vi "SCC-manual.vi"() -> (0 "vacuo 2":bool, 1 "vacuo (mBar)":dbl(knob) scale=0.0..1000.0, 2 "P02 (Bar)":dbl(knob) scale=0.0..20.0 scale format="%#_5g", 3 "P01 (Bar)":dbl(knob) scale=0.0..20.0, 4 "ATM 2":bool, 5 "Cam01 2":bool, 6 "Cam02 2":bool, 7 "Gas2":bool, 8 "T-02":dbl, 9 "T-01":dbl, 10 "Tc":dbl, 11 "Boolean":bool)   [LabVIEW 2011]
panel:
  in  "argument 7":dbl
  in  "argument 6":dbl
  in  "argument 5":dbl
  in  "argument 4":dbl
  in  "argument 3":dbl
  in  "argument 2":dbl
  in  "argument":dbl
  in  "Clear":bool
  out "Waveform Chart":T1(graph)
  in  "stop":bool
  out "Heat 2":bool
  out "Pelt 2":bool
  in  "Heat":bool
  in  "Pelt":bool
  in  "vacuo":bool
  in  "Gas":bool
  in  "ATM":bool
  in  "Cam02":bool
  in  "Cam01":bool
  # "Manual controller"
  # "Gas in"
  # "P - 01(bar)"
  # "P - 02(bar)"
  # "Cham-1"
  # "Cham-2"
  # "Atm"
  # "Tc"
  # "T-01"
  # "Vacuo"
  # "T-02"
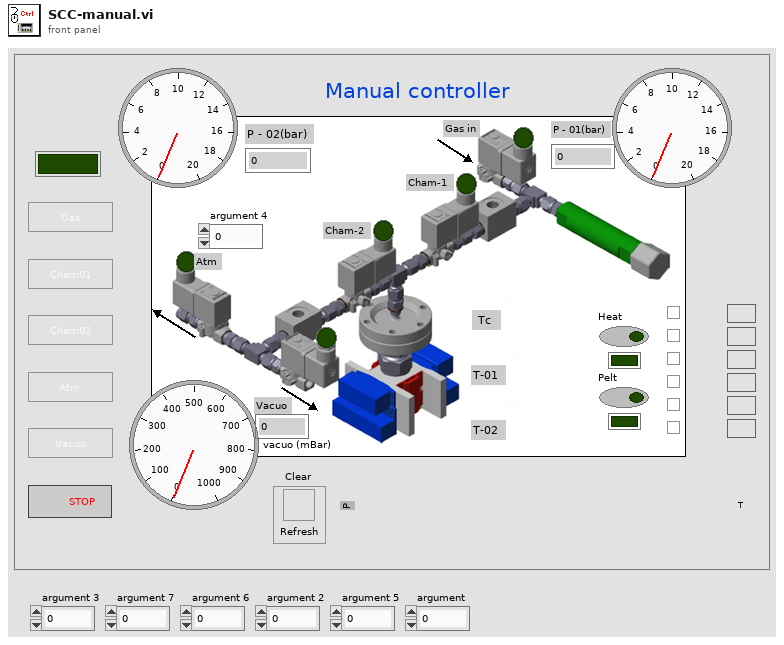
[diagram p1: front panel]
types:
  T1 = cluster{"P01 (Bar)":dbl, "P02 (Bar)":dbl, "vacuo (mBar)":dbl, "RTD-chamber (ºC)":sgl, "RTD-01 (ºC)":sgl, "RTD-02 (ºC)":sgl}
  T2 = cluster{"P01 (Bar)":dbl, "P02 (Bar)":dbl, "vacuo (mBar)":dbl, "RTD-chamber (ºC)":sgl, "RTD-01 (ºC)":sgl, "RTD-02 (ºC)":sgl}[]
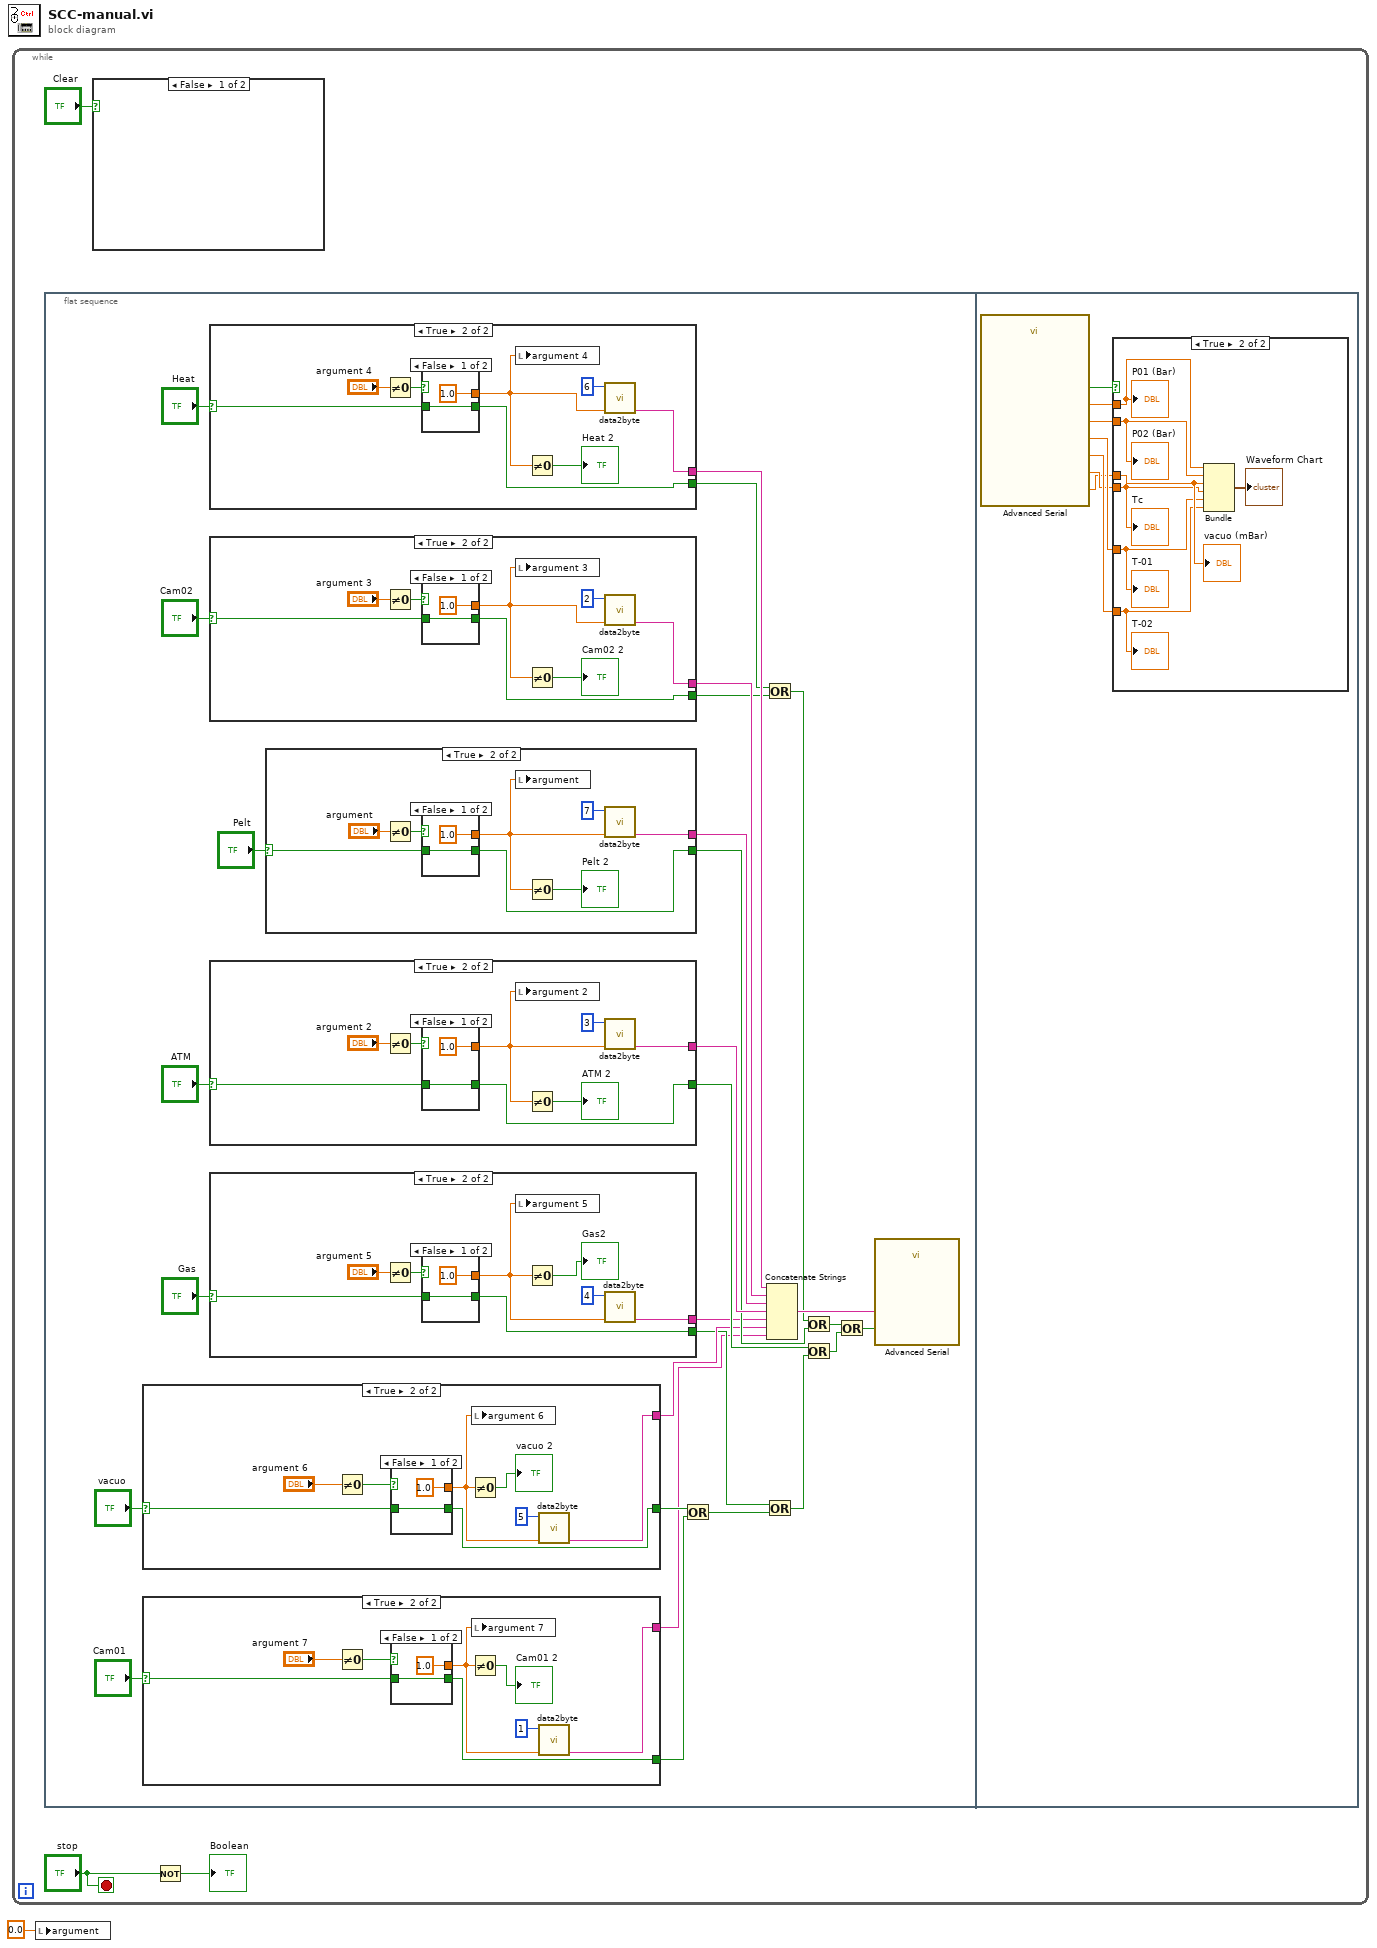
[diagram p0: block diagram]
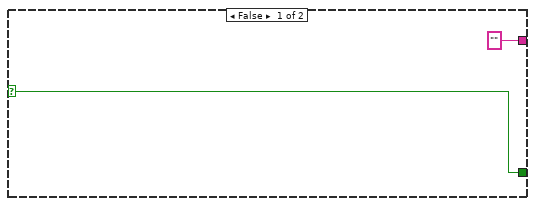
[diagram p2: hidden frame]
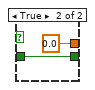
[diagram p3: hidden frame]
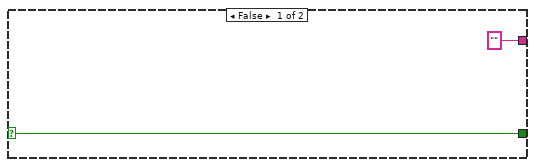
[diagram p4: hidden frame]
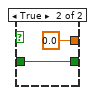
[diagram p5: hidden frame]
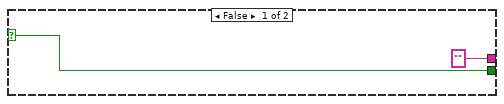
[diagram p6: hidden frame]
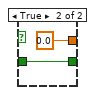
[diagram p7: hidden frame]
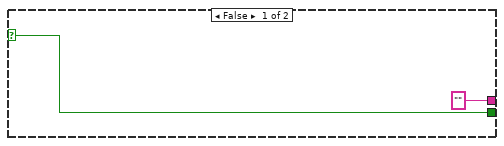
[diagram p8: hidden frame]
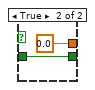
[diagram p9: hidden frame]
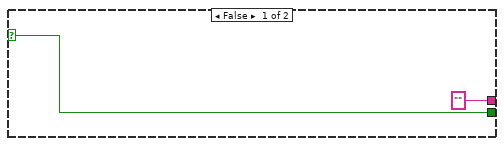
[diagram p10: hidden frame]
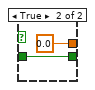
[diagram p11: hidden frame]
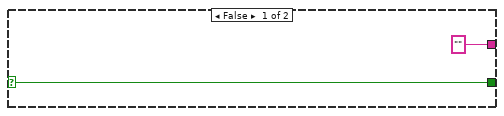
[diagram p12: hidden frame]
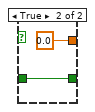
[diagram p13: hidden frame]
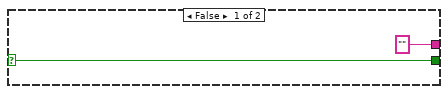
[diagram p14: hidden frame]
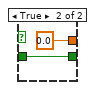
[diagram p15: hidden frame]
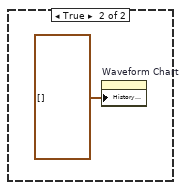
[diagram p17: hidden frame]
diagram:
  n1 = while {
    stop <- "stop" stop-if-true
    n2 = flat-sequence {
      frame #0 {
        n3 = case shown="True" "vacuo" {
          selector: "vacuo" -> [w47 w55]
          tunnel: [w47 w54] -> w7
          tunnel: ["" ("protocol") w50] -> w13
          frame False {
          }
          frame True {
            n4 = Not Equal To 0?(x="argument 6") -> (x != 0?=w56:bool)
            n5 = case shown="False" w56 {
              tunnel: [w58 w60] -> w54
              tunnel: w55 -> [w58 w60]
              tunnel: [1.0 ("number") 0.0 ("number")] -> w51
              frame False {
              }
              frame True {
              }
            }
            n6 = Not Equal To 0?(x=w51) -> (x != 0?=→"vacuo 2":bool)
            n7 = local write "argument 6"(w51) -> ()
            n8 = call "data2byte.vi"("argument"=w51, "new function"=5) -> ("protocol"=w50:string)  [unwired: 8 in, 1 out]
          }
        }
        n9 = case shown="True" "Cam01" {
          selector: "Cam01" -> [w33 w41]
          tunnel: [w33 w40] -> w9
          tunnel: ["" ("protocol") w36] -> w5
          frame False {
          }
          frame True {
            n10 = Not Equal To 0?(x="argument 7") -> (x != 0?=w42:bool)
            n11 = case shown="False" w42 {
              tunnel: [w44 w46] -> w40
              tunnel: w41 -> [w44 w46]
              tunnel: [1.0 ("number") 0.0 ("number")] -> w37
              frame False {
              }
              frame True {
              }
            }
            n12 = Not Equal To 0?(x=w37) -> (x != 0?=→"Cam01 2":bool)
            n13 = local write "argument 7"(w37) -> ()
            n14 = call "data2byte.vi"("argument"=w37, "new function"=1) -> ("protocol"=w36:string)  [unwired: 8 in, 1 out]
          }
        }
        n15 = case shown="True" "Heat" {
          selector: "Heat" -> [w75 w83]
          tunnel: [w75 w82] -> w20
          tunnel: ["" ("protocol") w78] -> w21
          frame False {
          }
          frame True {
            n16 = Not Equal To 0?(x="argument 4") -> (x != 0?=w84:bool)
            n17 = case shown="False" w84 {
              tunnel: [w86 w88] -> w82
              tunnel: w83 -> [w86 w88]
              tunnel: [1.0 ("number") 0.0 ("number")] -> w79
              frame False {
              }
              frame True {
              }
            }
            n18 = local write "argument 4"(w79) -> ()
            n19 = Not Equal To 0?(x=w79) -> (x != 0?=→"Heat 2":bool)
            n20 = call "data2byte.vi"("argument"=w79, "new function"=6) -> ("protocol"=w78:string)  [unwired: 8 in, 1 out]
          }
        }
        n21 = case shown="True" "Cam02" {
          selector: "Cam02" -> [w89 w97]
          tunnel: [w89 w96] -> w19
          tunnel: ["" ("protocol") w92] -> w26
          frame False {
          }
          frame True {
            n22 = Not Equal To 0?(x="argument 3") -> (x != 0?=w98:bool)
            n23 = case shown="False" w98 {
              tunnel: [w100 w102] -> w96
              tunnel: w97 -> [w100 w102]
              tunnel: [1.0 ("number") 0.0 ("number")] -> w93
              frame False {
              }
              frame True {
              }
            }
            n24 = local write "argument 3"(w93) -> ()
            n25 = Not Equal To 0?(x=w93) -> (x != 0?=→"Cam02 2":bool)
            n26 = call "data2byte.vi"("argument"=w93, "new function"=2) -> ("protocol"=w92:string)  [unwired: 8 in, 1 out]
          }
        }
        n27 = case shown="True" "ATM" {
          selector: "ATM" -> [w103 w111]
          tunnel: [w103 w110] -> w17
          tunnel: ["" ("protocol") w106] -> w28
          frame False {
          }
          frame True {
            n28 = Not Equal To 0?(x="argument 2") -> (x != 0?=w112:bool)
            n29 = case shown="False" w112 {
              tunnel: [w114 w116] -> w110
              tunnel: w111 -> [w114 w116]
              tunnel: [1.0 ("number") 0.0 ("number")] -> w107
              frame False {
              }
              frame True {
              }
            }
            n30 = local write "argument 2"(w107) -> ()
            n31 = Not Equal To 0?(x=w107) -> (x != 0?=→"ATM 2":bool)
            n32 = call "data2byte.vi"("argument"=w107, "new function"=3) -> ("protocol"=w106:string)  [unwired: 8 in, 1 out]
          }
        }
        n33 = case shown="True" "Gas" {
          selector: "Gas" -> [w61 w69]
          tunnel: [w61 w68] -> w12
          tunnel: ["" ("protocol") w64] -> w14
          frame False {
          }
          frame True {
            n34 = Not Equal To 0?(x="argument 5") -> (x != 0?=w70:bool)
            n35 = case shown="False" w70 {
              tunnel: [w72 w74] -> w68
              tunnel: w69 -> [w72 w74]
              tunnel: [1.0 ("number") 0.0 ("number")] -> w65
              frame False {
              }
              frame True {
              }
            }
            n36 = local write "argument 5"(w65) -> ()
            n37 = Not Equal To 0?(x=w65) -> (x != 0?=→"Gas2":bool)
            n38 = call "data2byte.vi"("argument"=w65, "new function"=4) -> ("protocol"=w64:string)  [unwired: 8 in, 1 out]
          }
        }
        n39 = case shown="True" "Pelt" {
          selector: "Pelt" -> [w117 w125]
          tunnel: [w117 w124] -> w25
          tunnel: ["" ("protocol") w119] -> w29
          frame False {
          }
          frame True {
            n40 = Not Equal To 0?(x="argument") -> (x != 0?=w126:bool)
            n41 = case shown="False" w126 {
              tunnel: [w128 w130] -> w124
              tunnel: w125 -> [w128 w130]
              tunnel: [1.0 ("number") 0.0 ("number")] -> w120
              frame False {
              }
              frame True {
              }
            }
            n42 = local write "argument"(w120) -> ()
            n43 = Not Equal To 0?(x=w120) -> (x != 0?=→"Pelt 2":bool)
            n44 = call "data2byte.vi"("argument"=w120, "new function"=7) -> ("protocol"=w119:string)  [unwired: 8 in, 1 out]
          }
        }
        n45 = Or(x=w7, y=w9) -> (x .or. y?=w6:bool)
        n46 = Or(x=w20, y=w19) -> (x .or. y?=w18:bool)
        n47 = Or(x=w12, y=w6) -> (x .or. y?=w11:bool)
        n48 = Concatenate Strings(w21, w26, w29, w28, w14, w13, w5) -> (w27:string)
        n49 = Or(x=w18, y=w25) -> (x .or. y?=w24:bool)
        n50 = Or(x=w17, y=w11) -> (x .or. y?=w16:bool)
        n51 = Or(x=w24, y=w16) -> (x .or. y?=w30:bool)
        n52 = call "Advanced Serial.vi"("Write"=w30, "string to write"=w27) -> ()  [unwired: 3 in, 7 out]
      }
      frame #1 {
        n53 = call "Advanced Serial.vi"() -> ("RTD-02 (ºC)"=w133:sgl, "RTD-01 (ºC)"=w135:sgl, "vacuo (mBar)"=w131:dbl, "P02 (Bar)"=w137:dbl, "RTD-chamber (ºC)"=w132:sgl, "P01 (Bar)"=w136:dbl, "32bytes"=w134:bool)  [unwired: 5 in]
        n54 = case shown="True" w134 {
          tunnel: w136 -> [_ w144]
          tunnel: w135 -> [_ w140]
          tunnel: w133 -> [_ w139]
          tunnel: w132 -> [_ w141]
          tunnel: w131 -> [_ w142]
          tunnel: w137 -> [_ w143]
          frame False {
          }
          frame True {
            n55 = Bundle("P01 (Bar)"=w144, "P02 (Bar)"=w143, "vacuo (mBar)"=w142, "RTD-chamber (ºC)"=w141, "RTD-01 (ºC)"=w140, "RTD-02 (ºC)"=w139) -> (→"Waveform Chart":T1)  [unwired: 1 in]
            "Tc" <- w141
            "T-01" <- w140
            "T-02" <- w139
            "P02 (Bar)" <- w143
            "P01 (Bar)" <- w144
            "vacuo (mBar)" <- w142
          }
        }
      }
    }
    n56 = case shown="False" "Clear" {
      frame False {
      }
      frame True {
        n57 = property on="Waveform Chart" class="WFChart (strict)"("History Data"=T2 []) -> ()  [unwired: 2 in, 2 out]
      }
    }
    n58 = Not(x="stop") -> (.not. x?=→"Boolean":bool)
  }
  n59 = local write "argument"(0.0 ("argument")) -> ()
